vi "Adjust Splitter.vi"(8 "error in":errorcluster, 9 "Show":bool, 10 "Splitter":cluster{"Splitter":refnum<vi>, "Initial":i32}, 11 "Right Panel in":refnum<class "Right.lvclass">) -> (0 "error out":errorcluster, 3 "Right Panel out":refnum<class "Right.lvclass">)   [LabVIEW 2023, in "Right.lvlib" / "Right.lvclass"]
uses:
  Project/Right.lvclass
  C:/Users/Public/Documents/Development/builds/Engine/Engine.lvlibp/Project/Engine.lvclass
  builds/Engine/Engine.lvlibp/Accessors/Read VI_Ref.vi
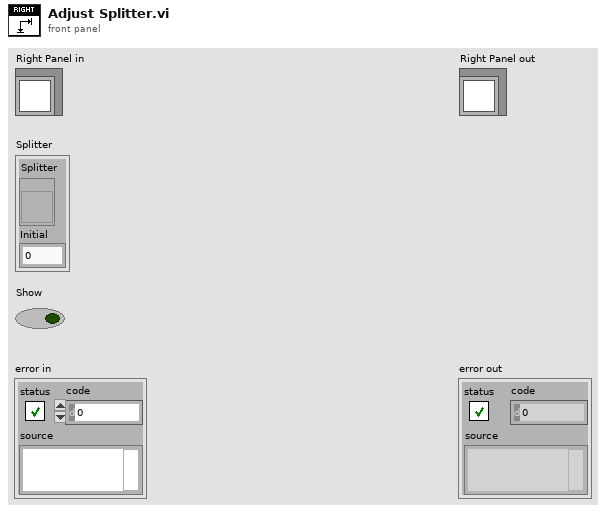
[diagram p1: front panel]
types:
  T1 = typedef "LVPointTypeDef.ctl" = cluster{"Horizontal":i16, "Vertical":i16}
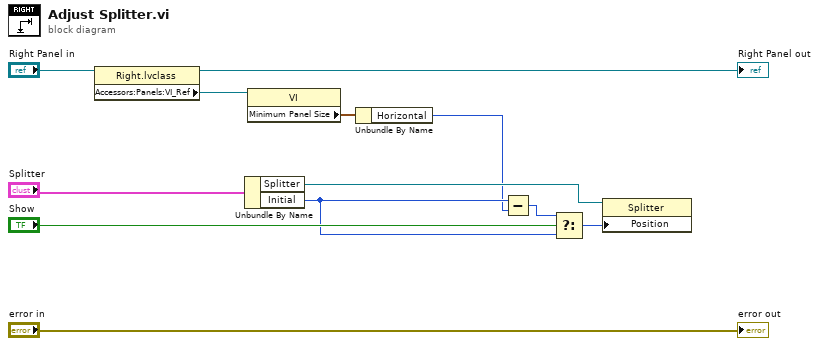
[diagram p0: block diagram]
diagram:
  n1 = property class="Right.lvclass"(reference="Right Panel in") -> (reference out=→"Right Panel out":refnum<class "Right.lvclass">, "Accessors:Panels:VI_Ref"=w2:refnum<vi>)  [unwired: 1 in, 1 out]
  n2 = Unbundle By Name("Splitter") -> ("Splitter"=w8:refnum<vi>, "Initial"=w5:i32)
  n3 = property class="VI"(reference=w2) -> ("Minimum Panel Size"=w9:T1)  [unwired: 1 in, 2 out]
  n4 = Unbundle By Name(w9) -> ("Horizontal"=w4:i16)
  n5 = Subtract(x=w5, y=w4) -> (x-y=w6:i32)
  n6 = Select(t=w6, s="Show", f=w5) -> (s? t:f=w7:i32)
  n7 = property class="Splitter"(reference=w8, "Position"=w7) -> ()  [unwired: 1 in, 2 out]
  "error out" <- "error in"
